vi "CaseSelector.vi"(6 "error in":errorcluster, 9 "CaseStructure in":refnum<class "CaseStructure.lvclass">) -> (0 "error out":errorcluster, 3 "CaseStructure out":refnum<class "CaseStructure.lvclass">, 4 "Selector.UID":i32)   [LabVIEW 2014, in "CaseStructure.lvclass"]
uses:
  CaseStructure.lvclass
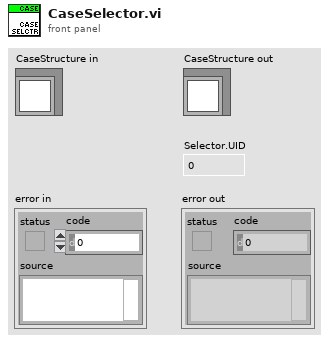
[diagram p1: front panel]
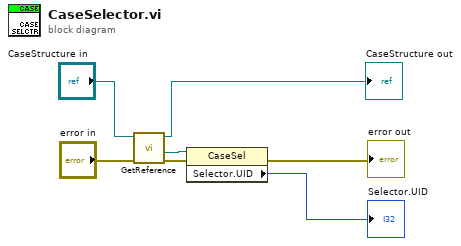
[diagram p0: block diagram]
diagram:
  n1 = call "GetReference.vi"("error in"="error in", "CaseStructure in"="CaseStructure in") -> ("error out"=w6:errorcluster, "reference out"=w7:refnum<vi>, "CaseStructure out"=→"CaseStructure out":refnum<class "CaseStructure.lvclass">)  [unwired: 7 in]
  n2 = property class="CaseSel"(reference=w7, error in=w6) -> (error out=→"error out":errorcluster, "Selector.UID"=→"Selector.UID":i32)  [unwired: 1 out]
